vi "nanocal -- nuclear schottky fit V8.vi"() -> ()   [LabVIEW 2021] (continued)
          }
          frame "action: update state of selectors" {
            w1061 = T1[] [enum."T (K)", enum."B (T)", enum."θ (deg)", enum."side (S|R)"] items=["ζ", "τ1", "τS", "τN", "τC", "κ0", "m1", "m2", "m3", "T (K)", "B (T)", "θ (deg)", "side (S|R)", "set of (B|T)", "Re(offset)", "Im(offset)", "στ1", "στ1-", "στ1+", "στS", "στS-", "στS+", "στN", "στN-", "στN+", "τ11", "τ12", "τ21", "τ22", "τN1", "τN2", "σηlogτ1", "σηlogτS", "σηlogτN", "σlogτ1", "σlogτS", "σlogτN", "σητ1", "σητS", "σητN", "noiseT"]  # selector fields
            n504 = local read "what?"() -> (w1057:T6)
            n505 = Unbundle By Name(w1057) -> ("side (8S|4R)"=w1056:i64, "ignore side !"=w1055:bool, "lookup.side lookup"=w1054:map{i32, dbl}, "T (K)"=w1051:dbl, "ignore T !"=w1053:bool, "lookup.T lookup"=w1052:map{i32, dbl}, "B (T)"=w1048:dbl, "ignore B !"=w1050:bool, "lookup.B lookup"=w1049:map{i32, dbl}, "θ (∘)"=w1046:dbl, "ignore θ !"=w1045:bool, "lookup.θ lookup"=w1047:map{i32, dbl}, "set (1T|2B)"=w1042:i32, "ignore set of !"=w1043:bool, "lookup.set of lookup"=w1044:map{i32, dbl})
            n506 = local read "new selector names"() -> (w1064:map{T1, map{T14, string}})
            n507 = Look In Map(map=w1054, key=w1056) -> (value=w1060:dbl)  [unwired: 1 in, 1 out]
            n508 = node(w1055, w1060) -> (w1081:map{bool, dbl})
            n509 = Look In Map(map=w1052, key=w1051) -> (value=w1080:dbl)  [unwired: 1 in, 1 out]
            n510 = Look In Map(map=w1049, key=w1048) -> (value=w1076:dbl)  [unwired: 1 in, 1 out]
            n511 = node(w1053, w1080) -> (w1078:map{bool, dbl})
            n512 = node(w1050, w1076) -> (w1075:map{bool, dbl})
            n513 = Look In Map(map=w1047, key=w1046) -> (value=w1074:dbl)  [unwired: 1 in, 1 out]
            n514 = node(w1045, w1074) -> (w1072:map{bool, dbl})
            n515 = Look In Map(map=w1044, key=w1042) -> (value=w1071:dbl)  [unwired: 1 in, 1 out]
            n516 = node(w1043, w1071) -> (w1069:map{bool, dbl})
            n517 = local read "side map from NUM"() -> (w1058:map{i32, T9})
            n518 = node(3-lorentzian-parameters."side (S|R)" ("Plost: sweep window"), w1081, 3-lorentzian-parameters."T (K)" ("Plost: sweep window"), w1078, 3-lorentzian-parameters."B (T)" ("Plost: sweep window"), w1075, 3-lorentzian-parameters."θ (deg)" ("Plost: sweep window"), w1072, 3-lorentzian-parameters."set of (B|T)" ("Plost: sweep window"), w1069) -> (w1041:map{T1, map{bool, dbl}})
            "state of all selectors" <- w1041
            n519 = for {
              tunnel: w1064 -> [w1086]
              shift-right: [w1089] -> w1062
              shift-left: "_" ("event data") -> [w1088]
              tunnel: w1061 -> [w1085] mode=indexing
              tunnel: w1041 -> [w1083]
              n520 = Look In Map(map=w1083, key=w1085) -> (value=w1091:map{bool, dbl})  [unwired: 1 in, 1 out]
              n521 = Look In Map(map=w1086, key=w1085) -> (value=w1084:map{T14, string})  [unwired: 1 in, 1 out]
              n522 = for {
                tunnel: w1091 -> [w1106] mode=indexing
                tunnel: [w1105] -> w1090
                tunnel: [w1104] -> w1087
                n523 = Unbundle(w1106) -> ("ignore side !"=w1105:bool, "number OUT"=w1104:dbl)
              }
              n524 = case shown="False" w1090 {
                tunnel: [w1102 w1103] -> w1089
                tunnel: w1088 -> [w1101 w1103]
                tunnel: w1087 -> [w1098 _]
                tunnel: w1084 -> [w1094 _]
                frame False {
                  n525 = Look In Map(map=w1094, key=nameformattingitem."units") -> (value=w1095:string)  [unwired: 1 in, 1 out]
                  n526 = Look In Map(map=w1094, key=nameformattingitem."prec") -> (value=w1092:string)  [unwired: 1 in, 1 out]
                  n527 = Format Value(format string=w1092, value (0)=w1098) -> (output string=w1097:string)  [unwired: 1 in]
                  n528 = Concatenate Strings(w1101, "_" ("event data"), w1097, w1095, "_" ("event data")) -> (w1102:string)
                }
                frame True {
                }
              }
            }
            "state of all selectors string" <- w1062
            n529 = Look In Map(map=w1058, key=w1060) -> (value=w1059:T9)  [unwired: 1 in, 1 out]
            n530 = local write "side"(w1059) -> ()
            n531 = Generate User Event(user event=w1065, event data cluster="action: replot colors" ("event data")) -> (user event out=w1066:refnum<user-event>)  [unwired: 2 in, 1 out]
            n532 = Generate User Event(user event=w1066, event data cluster="action: update constrained file selector" ("event data")) -> ()  [unwired: 2 in, 2 out]
          }
          frame "action: copy from math" {
            w1107 = map{T1, dbl} {}  # Size: 0
            w1125 = map{T1, bool} {}  # Size: 0
            n533 = local read "defaults selector"() -> (w1124:T5)
            n534 = local read "mathematica thing"() -> (w1130:map{string, map{T1, dbl}})
            n535 = for {
              shift-right: [w1148] -> w1123
              shift-left: w1125 -> [w1149]
              tunnel: w1124 -> [w1147] mode=indexing
              n536 = Unbundle(w1147) -> ("Plost: sweep window"=w1146:T1, "used default"=w1145:bool)
              n537 = Insert Into Map(map in=w1149, key=w1146, value=w1145) -> (map out=w1148:map{T1, bool})  [unwired: 2 out]
            }
            n538 = case shown="True" "overwrite \noffset" {
              selector: "overwrite \noffset" -> [w1139 w1141]
              tunnel: w1122 -> [w1140 w1144]
              tunnel: [w1140 w1143] -> w1115
              tunnel: w1117 -> [_ w1142]
              tunnel: [w1139 w1141] -> w1108
              frame False {
              }
              frame True {
                n539 = Build Array (concatenate)(w1144, w1142) -> (w1143:T1[])
              }
            }
            n540 = local read "key"() -> (w1129:string)
            n541 = local read "parameter map"() -> (w1120:map{T1, dbl})
            n542 = case shown="True" "overwrite noiseT" {
              selector: "overwrite noiseT" -> [w1131 w1133]
              tunnel: w1115 -> [w1132 w1136]
              tunnel: [w1132 w1135] -> w1116
              tunnel: w1114 -> [_ w1134]
              tunnel: [w1131 w1133] -> w1112
              frame False {
              }
              frame True {
                n543 = Build Array (concatenate)(w1136, w1134) -> (w1135:T1[])
              }
            }
            n544 = Look In Map(map=w1130, key=w1129) -> (key not found?=w1127:bool, value=w1128:map{T1, dbl})  [unwired: 1 in]
            n545 = case shown="False" w1127 {
              tunnel: w1128 -> [w1163 _]
              tunnel: w1123 -> [w1161 _]
              tunnel: w1116 -> [w1162 _]
              tunnel: w1108 -> [w1160 w1206]
              tunnel: [w1159 w1206] -> w1111
              tunnel: w1120 -> [w1158 _]
              tunnel: w1118 -> [w1157 _]
              tunnel: w1112 -> [w1154 w1205]
              tunnel: [w1153 w1205] -> w1110
              tunnel: w1107 -> [w1151 _]
              frame False {
                # "the order of numbers \nMUST corrspond to order\nin the \"parameter\" array"
                n546 = for {
                  tunnel: w1163 -> [w1197]
                  tunnel: w1162 -> [w1187] mode=indexing
                  tunnel: w1161 -> [w1196]
                  shift-right: [w1191] -> w1152
                  shift-left: w1158 -> [w1192]
                  shift-right: [w1188] -> w1150
                  shift-left: w1151 -> [w1189]
                  n547 = Look In Map(map=w1196, key=w1187, default value=FALSE) -> (value=w1195:bool)  [unwired: 1 out]
                  n548 = Look In Map(map=w1197, key=w1187, default value=0.0) -> (value=w1194:dbl)  [unwired: 1 out]
                  n549 = case shown="True" w1195 {
                    tunnel: w1194 -> [w1200 _]
                    tunnel: w1187 -> [_ w1202]
                    tunnel: [w1200 w1201] -> w1186
                    frame False {
                    }
                    frame True {
                      n550 = local read "T (K)"() -> (w1204:dbl)
                      n551 = call "nanocal -- defaut parameter manager -- V1.vi"("action"=nanocal_--_defaut_parameter_manager_action--_V1."get logarithmic interp", "T"=w1204, "what"=w1202) -> ("number"=w1201:dbl)  [unwired: 8 in]
                    }
                  }
                  n552 = Insert Into Map(map in=w1189, key=w1187, value=w1186) -> (map out=w1188:map{T1, dbl})  [unwired: 2 out]
                  n553 = in-place {
                    in-place-border: w1186 -> [w1199]
                    in-place-border: LVMapReplaceAction."Modify Entry only if found" ("action") -> [w1198]
                    n554 = in-place-map #5(w1192, w1187) -> ()  [unwired: 1 in, 2 out]
                    n555 = in-place-map #5(w1199, w1198) -> (w1191:map{T1, dbl})  [unwired: 2 out]
                  }
                }
                n556 = case shown="True" w1154 {
                  selector: w1154 -> [w1164 w1170]
                  tunnel: [w1164 w1170] -> w1153
                  tunnel: w1150 -> [_ w1168]
                  frame False {
                  }
                  frame True {
                    n557 = local read "errors&stuff"() -> (w1167:T10)
                    n558 = Look In Map(map=w1168, key=3-lorentzian-parameters."noiseT" ("x")) -> (value=w1166:dbl)  [unwired: 1 in, 1 out]
                    n559 = in-place {
                      in-place-border: w1166 -> [w1171]
                      n560 = in-place-cluster #6(w1167) -> ()  [unwired: 1 out]
                      n561 = in-place-cluster #6("noise T"=w1171) -> (w1165:T10)
                    }
                    n562 = local write "errors&stuff"(w1165) -> ()
                  }
                }
                n563 = case shown="True" w1160 {
                  selector: w1160 -> [w1177 w1184]
                  tunnel: [w1177 w1184] -> w1159
                  tunnel: w1150 -> [_ w1183]
                  frame False {
                  }
                  frame True {
                    n564 = Look In Map(map=w1183, key=3-lorentzian-parameters."Im(offset)" ("x")) -> (value=w1179:dbl)  [unwired: 1 in, 1 out]
                    n565 = Look In Map(map=w1183, key=3-lorentzian-parameters."Re(offset)" ("x")) -> (value=w1180:dbl)  [unwired: 1 in, 1 out]
                    n566 = Bundle("number OUT"=w1180, "number OUT"=w1179) -> (w1178:cluster{"number OUT":dbl, "number OUT":dbl})  [unwired: 1 in]
                    n567 = local write "offset Re\noffset Im"(w1178) -> ()
                  }
                }
                n568 = flat-sequence {
                  tunnel: w1152 -> [w1172]
                  tunnel: w1157 -> [w1176]
                  tunnel: "interface: update list from parameter map" ("event data") -> [w1175]
                  tunnel: "interface: update curvature plot" ("event data") -> [w1173]
                  frame #0 {
                    n569 = local write "parameter map"(w1172) -> ()
                  }
                  frame #1 {
                    n570 = Generate User Event(user event=w1176, event data cluster=w1175) -> (user event out=w1174:refnum<user-event>)  [unwired: 2 in, 1 out]
                    n571 = Generate User Event(user event=w1174, event data cluster=w1173) -> ()  [unwired: 2 in, 2 out]
                  }
                }
              }
              frame True {
              }
            }
            n572 = Or(x=w1111, y=w1110) -> (x .or. y?=w1109:bool)
            n573 = case shown="True" w1109 {
              tunnel: ["action: new sweep" ("event data") "action: read from file" ("event data")] -> w1119
              frame False {
              }
              frame True {
              }
            }
            n574 = Generate User Event(user event=w1126, event data cluster=w1119) -> ()  [unwired: 2 in, 2 out]
          }
          frame "action: copy to math" {
            n575 = local read "newton parameters"() -> (w1228:T2)
            n576 = local read "error weights"() -> (w1227:T4)
            n577 = local read "parameter map"() -> (w1217:map{T1, dbl})
            n578 = local read "errors&stuff"() -> (w1211:T10)
            n579 = call "nanocal -- publish -- freq scan V2.vi"("publisher action"=publisher_action."get") -> ("data"=w1218:T21)  [unwired: 7 in, 3 out]
            n580 = Bundle By Name(cluster=w1228, "weighting"=w1227) -> (w1219:T2)
            n581 = Generate User Event(user event=w1241, event data cluster="action: replot colors" ("event data")) -> ()  [unwired: 2 in, 2 out]
            n582 = call "nanocal -- generate 3D curvature ellipsoid --  V5.vi"("parameter keys IN"=w1216, "parameter tensor order IN"=w1215, "parameters IN"=w1217, "data IN"=w1218, "errors IN"=w1211, "newton parameters"=w1219) -> ("errors pair OUT"=w1209:T10)  [unwired: 9 in]
            n583 = Build Array (concatenate)(w1220, w1222, w1208, w1207) -> (w1221:T1[])
            n584 = Unbundle By Name(w1209) -> ("pars & errors"=w1223:map{T1, dbl})
            n585 = local write "errors&stuff"(w1209) -> ()
            n586 = local read "offset Re\noffset Im"() -> (w1231:cluster{"Numeric":dbl, "Numeric":dbl})
            n587 = local read "θ (deg)"() -> (w1235:dbl)
            n588 = for {
              tunnel: w1222 -> [w1245] mode=indexing
              shift-right: [w1246] -> _
              shift-left: w1223 -> [w1246]
              tunnel: [w1244] -> w1225 mode=indexing
              n589 = Look In Map(map=w1246, key=w1245, default value=0.0) -> (value=w1244:dbl)  [unwired: 1 out]
            }
            n590 = local read "T (K)"() -> (w1237:dbl)
            n591 = local read "B (T)"() -> (w1236:dbl)
            n592 = Unbundle(w1231) -> ("Numeric"=w1214:dbl, "Numeric"=w1213:dbl)
            n593 = Unbundle By Name(w1209) -> ("noise T"=w1210:dbl)
            n594 = local read "parameter map"() -> (w1230:map{T1, dbl})
            n595 = Build Array(w1214, w1213) -> (w1212:dbl[])
            n596 = Build Array(w1237, w1236, w1235) -> (w1226:dbl[])
            n597 = Build Array (concatenate)(w1226, w1225, w1212, w1210) -> (w1224:dbl[])
            n598 = for {
              tunnel: w1224 -> [w1247] mode=indexing
              tunnel: w1221 -> [w1248] mode=indexing
              shift-right: [w1249] -> w1234
              shift-left: w1230 -> [w1250]
              n599 = Insert Into Map(map in=w1250, key=w1248, value=w1247) -> (map out=w1249:map{T1, dbl})  [unwired: 2 out]
            }
            n600 = local read "mathematica thing"() -> (w1240:map{string, map{T1, dbl}})
            n601 = local read "key"() -> (w1239:string)
            n602 = call "3-lorentzian-heat-response -- V4.vi"("action"=3-lorentzian-heat-response_action."calc m1m2m3", "Map IN"=w1234) -> ("Map OUT"=w1233:map{T1, dbl})  [unwired: 7 in, 2 out]
            n603 = in-place {
              in-place-border: w1233 -> [w1251]
              n604 = in-place-map #7(w1240, w1239) -> (w1254:map{T1, dbl})  [unwired: 1 in, 1 out]
              n605 = for {
                tunnel: w1251 -> [w1256] mode=indexing
                shift-right: [w1259] -> w1253
                shift-left: w1254 -> [w1260]
                shift-right: [w1258] -> _
                shift-left: w1251 -> [w1258]
                n606 = Unbundle(w1256) -> ("X selector"=w1255:T1)  [unwired: 1 out]
                n607 = Look In Map(map=w1258, key=w1255) -> (value=w1257:dbl)  [unwired: 1 in, 1 out]
                n608 = Insert Into Map(map in=w1260, key=w1255, value=w1257) -> (map out=w1259:map{T1, dbl})  [unwired: 2 out]
              }
              n609 = in-place-map #7(w1253, LVMapReplaceAction."Modify Entry only if found" ("action")) -> (w1238:map{string, map{T1, dbl}})  [unwired: 2 out]
            }
            n610 = local write "mathematica thing"(w1238) -> ()
          }
          frame "action: exit" {
          }
          frame "action: read from file" {
            n611 = local read "Read from file"() -> (w1269:path)
            n612 = Unbundle("offset Re\noffset Im") -> ("Numeric"=w1295:dbl, "Numeric"=w1294:dbl)
            n613 = Re/Im To Complex(1:w1294, 2:w1295) -> (0:w1282:cdb)
            n614 = call "file - read-write - list of lines-V2.vi"("read/write control"=file_--_read-write_control."read", "file path"=w1269) -> ("header OUT"=w1279:string, "list of lines OUT"=w1281:string[], "filename out"=w1309:string)  [unwired: 7 in]
            n615 = local read "cursor x selector"() -> (w1292:map{T1, dbl})
            n616 = call "filename-manage.vi"("filename-action"=filename-action."get name", "file name IN"=w1309) -> ("string OUT"=w1278:string)  [unwired: 7 in, 2 out]
            n617 = call "filename-manage.vi"("filename-action"=filename-action."get T", "file name IN"=w1278) -> ("number OUT"=w1291:dbl, "filename OUT"=w1306:string)  [unwired: 7 in, 1 out]
            "T (K)" <- w1291
            n618 = case shown="\"raw nanocal\"" "data file formatting" {
              tunnel: [w1318 w1345 w1394 w1421] -> w1303
              tunnel: [w1317 w1344 w1393 w1420] -> w1297
              tunnel: w1282 -> [w1316 w1339 w1389 w1410]
              tunnel: w1281 -> [w1319 w1353 w1388 w1409]
              tunnel: w1279 -> [_ w1354 _ _]
              tunnel: w1278 -> [_ w1351 _ _]
              tunnel: w1269 -> [_ w1352 _ _]
              tunnel: "side" -> [_ w1350 _ _]
              tunnel: "toggle generate labview files" -> [_ w1348 _ _]
              tunnel: "apply RC transform" -> [_ w1332 _ _]
              frame "as is", Default {
                n619 = for {
                  tunnel: w1319 -> [w1330] mode=indexing
                  tunnel: [w1325] -> w1320 mode=indexing if=w1321
                  tunnel: [w1324] -> w1318 mode=indexing if=w1321
                  w1326 = 0.0
                  n620 = Scan From String(format string="%f%f%f", input string=w1330, initial scan location=u32 0, default 1=w1326, default 2=w1326, default 3=w1326) -> (offset past scan=w1322:u32, output 1=w1324:dbl, output 2=w1328:dbl, output 3=w1327:dbl)  [unwired: 1 in, 2 out]
                  n621 = Greater Than 0?(x=w1322) -> (x > 0?=w1321:bool)
                  n622 = Re/Im To Complex(1:w1327, 2:w1328) -> (0:w1325:cdb)
                }
                n623 = Subtract(x=w1320, y=w1316) -> (x-y=w1317:cdb[])
              }
              frame "raw nanocal" {
                (unwired) array_--_freq-voltage_transformations_action."add -ω" ("freq voltage action")
                w1347 = T29[] [enum."add -ω", enum."sort ω", enum."select |ω|<max"] items=["as is", "add -ω", "sort ω", "2 x ω", "R-phase(deg) to Re-Im", "select ω>0", "labview file str", "select |ω|<max", "apply RC transform", "subtract background"]
                n624 = case shown="\"ref\"" w1350 {
                  tunnel: [nanocal_raw_file_manage_action_V1."read S side" ("action") nanocal_raw_file_manage_action_V1."read R side" ("action")] -> w1349
                  frame "sam", Default {
                  }
                  frame "ref" {
                  }
                }
                n625 = call "nanocal_raw_file_manage_V1.vi"("action"=w1349, "list of lines IN"=w1353, "header IN"=w1354) -> ("z (K/W)  OUT"=w1338:cdb[], "f (Hz) OUT"=w1341:dbl[], "correct temperature"=→"correct temperature":dbl)  [unwired: 5 in, 1 out]
                n626 = call "array -- freq-voltage transformations.vi"("number"=w1339, "freq voltage action"=array_--_freq-voltage_transformations_action."subtract background", "z In"=w1338, "ω IN"=w1341) -> ("z out"=w1336:cdb[], "ω out"=w1340:dbl[])  [unwired: 4 in, 2 out]
                n627 = case shown="True" w1332 {
                  tunnel: w1340 -> [w1356 w1363]
                  tunnel: [w1356 w1362] -> w1337
                  tunnel: w1336 -> [w1355 w1361]
                  tunnel: [w1355 w1360] -> w1335
                  tunnel: "tau" -> [_ w1359]
                  tunnel: array_--_freq-voltage_transformations_action."apply RC transform" ("freq voltage action") -> [_ w1358]
                  tunnel: "alpha" -> [_ w1357]
                  frame False {
                  }
                  frame True {
                    n628 = call "array -- freq-voltage transformations.vi"("number"=w1359, "freq voltage action"=w1358, "alpha"=w1357, "z In"=w1361, "ω IN"=w1363) -> ("z out"=w1360:cdb[], "ω out"=w1362:dbl[])  [unwired: 3 in, 2 out]
                  }
                }
                n629 = for {
                  shift-right: [w1367] -> w1345
                  shift-left: w1337 -> [w1368]
                  shift-right: [w1366] -> w1344
                  shift-left: w1335 -> [w1369]
                  tunnel: w1347 -> [w1365] mode=indexing
                  tunnel: "|ω| < limit (Hz)" -> [w1364]
                  n630 = call "array -- freq-voltage transformations.vi"("number"=w1364, "freq voltage action"=w1365, "z In"=w1369, "ω IN"=w1368) -> ("z out"=w1366:cdb[], "ω out"=w1367:dbl[])  [unwired: 4 in, 2 out]
                }
                n631 = case shown="True" w1348 {
                  tunnel: w1352 -> [_ w1381]
                  tunnel: w1351 -> [_ w1385]
                  tunnel: w1345 -> [_ w1377]
                  tunnel: w1344 -> [_ w1376]
                  frame False {
                  }
                  frame True {
                    n632 = call "filename-manage.vi"("filename-action"=filename-action."get basename", "file name IN"=w1385) -> ("string OUT"=w1383:string)  [unwired: 7 in, 2 out]
                    n633 = Strip Path(path=w1381) -> (stripped path=w1380:path)  [unwired: 1 out]
                    n634 = Concatenate Strings(w1383, "_labview_.dat") -> (w1372:string)
                    n635 = call "array -- freq-voltage transformations.vi"("freq voltage action"=array_--_freq-voltage_transformations_action."labview file str", "z In"=w1376, "ω IN"=w1377) -> ("lines out"=w1374:string[], "header OUT"=w1375:string)  [unwired: 5 in, 2 out]
                    n636 = Build Path(base path=w1380, name or relative path=w1372) -> (appended path=w1379:path)
                    n637 = call "file - read-write - list of lines-V2.vi"("read/write control"=file_--_read-write_control."write all", "header IN"=w1375, "list of lines IN"=w1374, "file path"=w1379) -> ()  [unwired: 5 in, 3 out]
                  }
                }
              }
              frame "add - ω" {
                n638 = for {
                  tunnel: w1388 -> [w1406] mode=indexing
                  tunnel: [w1401] -> w1390 mode=indexing if=w1397
                  tunnel: [w1400] -> w1386 mode=indexing if=w1397
                  w1402 = 0.0
                  n639 = Scan From String(format string="%f%f%f", input string=w1406, initial scan location=u32 0, default 1=w1402, default 2=w1402, default 3=w1402) -> (offset past scan=w1398:u32, output 1=w1400:dbl, output 2=w1404:dbl, output 3=w1403:dbl)  [unwired: 1 in, 2 out]
                  n640 = Greater Than 0?(x=w1398) -> (x > 0?=w1397:bool)
                  n641 = Re/Im To Complex(1:w1403, 2:w1404) -> (0:w1401:cdb)
                }
                n642 = Subtract(x=w1390, y=w1389) -> (x-y=w1387:cdb[])
                n643 = call "array -- freq-voltage transformations.vi"("freq voltage action"=array_--_freq-voltage_transformations_action."add -ω", "z In"=w1387, "ω IN"=w1386) -> ("z out"=w1395:cdb[], "ω out"=w1396:dbl[])  [unwired: 5 in, 2 out]
                n644 = call "array -- freq-voltage transformations.vi"("freq voltage action"=array_--_freq-voltage_transformations_action."sort ω", "z In"=w1395, "ω IN"=w1396) -> ("z out"=w1393:cdb[], "ω out"=w1394:dbl[])  [unwired: 5 in, 2 out]
              }
              frame "full rydh" {
                n645 = for {
                  tunnel: w1409 -> [w1433] mode=indexing
                  tunnel: [w1428] -> w1411 mode=indexing if=w1424
                  tunnel: [w1427] -> w1407 mode=indexing if=w1424
                  w1429 = 0.0
                  n646 = Scan From String(format string="%f%f%f", input string=w1433, initial scan location=u32 0, default 1=w1429, default 2=w1429, default 3=w1429) -> (offset past scan=w1425:u32, output 1=w1427:dbl, output 2=w1431:dbl, output 3=w1430:dbl)  [unwired: 1 in, 2 out]
                  n647 = Greater Than 0?(x=w1425) -> (x > 0?=w1424:bool)
                  n648 = Re/Im To Complex(1:w1430, 2:w1431) -> (0:w1428:cdb)
                }
                n649 = Subtract(x=w1411, y=w1410) -> (x-y=w1408:cdb[])
                n650 = call "array -- freq-voltage transformations.vi"("freq voltage action"=array_--_freq-voltage_transformations_action."2 x ω", "z In"=w1408, "ω IN"=w1407) -> ("z out"=w1415:cdb[], "ω out"=w1417:dbl[])  [unwired: 5 in, 2 out]
                n651 = call "array -- freq-voltage transformations.vi"("freq voltage action"=array_--_freq-voltage_transformations_action."R-phase(deg) to Re-Im", "z In"=w1415, "ω IN"=w1417) -> ("z out"=w1414:cdb[], "ω out"=w1416:dbl[])  [unwired: 5 in, 2 out]
                n652 = call "array -- freq-voltage transformations.vi"("freq voltage action"=array_--_freq-voltage_transformations_action."add -ω", "z In"=w1414, "ω IN"=w1416) -> ("z out"=w1422:cdb[], "ω out"=w1423:dbl[])  [unwired: 5 in, 2 out]
                n653 = call "array -- freq-voltage transformations.vi"("freq voltage action"=array_--_freq-voltage_transformations_action."sort ω", "z In"=w1422, "ω IN"=w1423) -> ("z out"=w1420:cdb[], "ω out"=w1421:dbl[])  [unwired: 5 in, 2 out]
              }
            }
            n654 = Insert Into Map(map in=w1292, key=3-lorentzian-parameters."T (K)" ("Plost: sweep window"), value=w1291) -> (map out=w1290:map{T1, dbl})  [unwired: 2 out]
            n655 = call "filename-manage.vi"("filename-action"=filename-action."get deg", "file name IN"=w1306) -> ("number OUT"=w1287:dbl, "filename OUT"=w1273:string)  [unwired: 7 in, 1 out]
            "θ (deg)" <- w1287
            n656 = Insert Into Map(map in=w1290, key=3-lorentzian-parameters."θ (deg)" ("Plost: sweep window"), value=w1287) -> (map out=w1289:map{T1, dbl})  [unwired: 2 out]
            n657 = call "filename-manage.vi"("filename-action"=filename-action."get B", "file name IN"=w1273) -> ("number OUT"=w1286:dbl, "filename OUT"=w1272:string)  [unwired: 7 in, 1 out]
            "B (T)" <- w1286
            n658 = Insert Into Map(map in=w1289, key=3-lorentzian-parameters."B (T)" ("Plost: sweep window"), value=w1286) -> (map out=w1288:map{T1, dbl})  [unwired: 2 out]
            n659 = local read "side map to STR"() -> (w1271:map{T9, string})
            n660 = local write "cursor x selector"(w1288) -> ()
            n661 = call "filename-manage.vi"("filename-action"=filename-action."getIDStock", "file name IN"=w1272) -> ("string OUT"=w1276:string)  [unwired: 7 in, 2 out]
            "file IDS" <- w1276
            n662 = Look In Map(map=w1271, key="side") -> (value=w1277:string)  [unwired: 1 in, 1 out]
            n663 = Concatenate Strings(w1276, w1277) -> (→"key":string)
            n664 = local read "folder"() -> (w1268:path)
            n665 = Build Path(base path=w1268, name or relative path=path "PLOTME.dat") -> (appended path=w1266:path)
            n666 = call "filter - complex - four.vi"("omega (Hz) in"=w1303, "z in"=w1297, "span"="cspan") -> ("omega out"=w1302:dbl[], "z out"=w1301:cdb[], "dz/domega out"=w1300:cdb[])  [unwired: 9 in, 5 out]
            n667 = call <vilib>:"Check if File or Folder Exists.vi"("path"=w1266) -> ("file or folder exists?"=w1265:bool, "dup path"=w1264:path)  [unwired: 8 in, 1 out]
            n668 = call "nanocal -- publish -- freq scan V2.vi"("publisher action"=publisher_action."set", "dz/dω IN (V)"=w1300, "z IN (V)"=w1301, "ω IN (Hz)"=w1302) -> ()  [unwired: 4 in, 4 out]
            n669 = case shown="True" w1265 {
              tunnel: w1264 -> [_ w1315]
              tunnel: [map{string, dbl[]} {} ("waves OUT") w1314] -> w1263
              frame False {
              }
              frame True {
                n670 = call "read waves - -V1.vi"("file path"=w1315) -> ("waves OUT"=w1314:map{string, dbl[]})  [unwired: 10 in]
              }
            }
            n671 = Generate User Event(user event=w1310, event data cluster="action: new sweep" ("event data")) -> ()  [unwired: 2 in, 2 out]
            n672 = local write "plotme waves"(w1263) -> ()
          }
          frame "action: save freq scan" {
            n673 = local read "Freq sweep name template"() -> (w1439:T8)
            n674 = call "MFLI -- publish -- freq scan.vi"("publisher action"=publisher_action."get") -> ("Voltage out (V)"=w1435:cdb[], "Freq out (Hz)"=w1436:dbl[])  [unwired: 9 in]
            n675 = call "filename-manage.vi"("filename pattern"=w1439, "filename-action"=filename-action."uniquenum", "folder IN"="Save folder", "file name IN"="freq sweep file name") -> ("filename OUT"=w1438:string)  [unwired: 5 in, 2 out]
            n676 = call "KM_appendline -- freq sweep.vi"("freq"=w1436, "Vout(V)"=w1435, "Save frequency scan"="Save folder", "read/write control"=KM_file_--_read-write_control."append one line", "name or relative path"=w1438) -> ()  [unwired: 15 in]
            n677 = local write "freq sweep file name"(w1438) -> ()
          }
          frame "void", Default {
          }
        }
      }
    }
  }
  n678 = while "interface events" {
    tunnel: w18 -> [w1447]
    tunnel: w45 -> [w1446]
    tunnel: w42 -> [w1445]
    tunnel: w19 -> [w1444]
    stop <- FALSE stop-if-true
    n679 = event shown="[10] \"alpha\", \"|ω| < limit (Hz)\", \"cspan\", \"tau\", \"apply RC transform\", \"offset Re offset Im\": Value Change" {
      selector: _ -> [_ _ _ _ _ _ _ _ _ _ _ _ _ _ _ _ _ _ _ _ _ _ _ _ _ _]
      dyn-events: _ -> [_ _ _ _ _ _ _ _ _ _ _ _ _ _ _ _ _ _ _ _ _ _ _ _ _ _]
      timeout: _ -> [_ _ _ _ _ _ _ _ _ _ _ _ _ _ _ _ _ _ _ _ _ _ _ _ _ _]
      tunnel: w1447 -> [w1448 _ w1461 w1485 _ w1510 w1516 _ w1520 w1522 w1524 w1527 w1533 _ w1627 w1648 w1668 w1670 w1674 w1677 w1680 w1683 w1691 w1695 w1697 w1700]
      tunnel: [_ _ _ _ _ _ _ _ "load! :l" _ _ _ _ _ _ _ _ _ _ _ _ _ _ _ _ _] -> _
      tunnel: [_ _ _ _ _ "go / pause!" _ _ _ _ _ "parse! :p" _ _ _ _ "Math→τ! :q" _ "τ→Math! :p" "Math→ string OUT! :s" "generate empty string from filelist !" "string IN → Math! :~" _ _ "plot landscape!" _] -> _
      tunnel: w1446 -> [_ w1452 _ _ w1487 _ _ _ _ _ _ _ w1529 _ _ _ _ _ _ _ _ _ _ _ _ _]
      tunnel: w1445 -> [_ _ _ _ _ _ _ _ _ _ _ _ _ _ w1635 w1656 _ _ _ _ _ _ _ _ _ _]
      tunnel: [_ _ _ _ _ _ _ _ _ "Read from file" _ _ _ _ _ _ _ _ _ _ _ _ _ _ _ _] -> _
      tunnel: [_ _ _ _ _ _ _ _ _ _ _ _ _ _ _ _ _ "load defaults" _ _ _ _ _ _ _ _] -> _
      tunnel: w1444 -> [_ _ w1463 _ _ _ _ _ _ _ _ _ _ w1622 w1625 w1646 _ _ _ _ _ _ _ _ _ _]
      event "Plot: circles": Cursor Move {
        n680 = event-data() -> ("CursIdx"=w1449:i32)  [unwired: 1 in]
        n681 = case shown="0..2" w1449 {
          tunnel: w1448 -> [w1451 _]
          frame 0..2 {
            w1450 = "action: fit"  # action
            n682 = Generate User Event(user event=w1451, event data cluster=w1450) -> ()  [unwired: 2 in, 2 out]
          }
          frame 3..5, Default {
          }
        }
      }
      event "scale gauge: Plot: circles": Value Change {
        n683 = event-data() -> ()  [unwired: 1 in, 1 out]
        n684 = local read "scale gauge: Plot: circles"() -> (w1458:dbl)
        n685 = Multiply(x=w1458, y=0.3) -> (x*y=w1459:dbl)
        n686 = Bundle By Name(cluster=T35 {"window y"=0.0021014740628288917, "center x"=44850.89441339177, "center y"=2.5658109925320947, "window x"=17480.201988350764} ("window IN"), "window x"=w1458, "window y"=w1458, "center x"=w1459, "center y"=0.0) -> (w1457:T35)
        n687 = call "replace cursor - plot ref - V2.vi"("Plot ref in"=w1452, "window IN"=w1457, "cursor action"=cursor_action."zoom to win") -> ()  [unwired: 13 in, 4 out]
      }
      event "ζ", "T1", "τS", "τN", "τC", "κ0": Value Change {
        w1464 = T1[] [enum."ζ", enum."τ1", enum."τS", enum."τN", enum."τC", enum."κ0"] items=["ζ", "τ1", "τS", "τN", "τC", "κ0", "m1", "m2", "m3", "T (K)", "B (T)", "θ (deg)", "side (S|R)", "set of (B|T)", "Re(offset)", "Im(offset)", "στ1", "στ1-", "στ1+", "στS", "στS-", "στS+", "στN", "στN-", "στN+", "τ11", "τ12", "τ21", "τ22", "τN1", "τN2", "σηlogτ1", "σηlogτS", "σηlogτN", "σlogτ1", "σlogτS", "σlogτN", "σητ1", "σητS", "σητN", "noiseT"]
        n688 = event-data() -> ()  [unwired: 1 in, 1 out]
        n689 = local read "τN"() -> (w1470:dbl)
        n690 = local read "τC"() -> (w1469:dbl)
        n691 = local read "κ0"() -> (w1468:dbl)
        n692 = local read "T1"() -> (w1472:dbl)
        n693 = local read "τS"() -> (w1471:dbl)
        n694 = local read "ζ"() -> (w1473:dbl)
        n695 = local read "parameter map"() -> (w1465:map{T1, dbl})
        n696 = Build Array(w1473, w1472, w1471, w1470, w1469, w1468) -> (w1467:dbl[])
        n697 = for {
          tunnel: w1464 -> [w1479] mode=indexing
          shift-right: [w1484] -> _
          shift-left: w1467 -> [w1484]
          shift-right: [w1481] -> w1466
          shift-left: w1465 -> [w1482]
          i -> [w1483]
          n698 = Index Array(array=w1484, index=w1483) -> (element=w1480:dbl)
          n699 = Insert Into Map(map in=w1482, key=w1479, value=w1480) -> (map out=w1481:map{T1, dbl})  [unwired: 2 out]
        }
        n700 = flat-sequence {
          tunnel: w1466 -> [w1474]
          tunnel: w1463 -> [w1478]
          tunnel: "interface: update color cursors" ("event data") -> [w1477]
          tunnel: w1461 -> [w1476]
          tunnel: "action: replot circles" ("event data") -> [w1475]
          frame #0 {
            n701 = local write "parameter map"(w1474) -> ()
          }
          frame #1 {
            n702 = Generate User Event(user event=w1476, event data cluster=w1475) -> ()  [unwired: 2 in, 2 out]
            n703 = Generate User Event(user event=w1478, event data cluster=w1477) -> ()  [unwired: 2 in, 2 out]
          }
        }
      }
      event Value Change {
        n704 = event-data() -> ()  [unwired: 1 in, 6 out]
        n705 = Generate User Event(user event=w1485, event data cluster="action: update enums" ("event data")) -> ()  [unwired: 2 in, 2 out]
      }
      event "ω0 (rad/sec)": Value Change {
        n706 = event-data() -> ()  [unwired: 1 in, 1 out]
        n707 = local read "parameter map"() -> (w1489:map{T1, dbl})
        n708 = call "nanocal -- publish -- freq scan V2.vi"("publisher action"=publisher_action."get") -> ("z out (V)"=w1507:cdb[], "ω out (Hz)"=w1502:dbl[])  [unwired: 7 in, 2 out]
        n709 = Divide(x="ω0 (rad/sec)", y=6.283185307179586) -> (x/y=w1500:dbl)
        n710 = call "3-lorentzian-heat-response -- V4.vi"("action"=3-lorentzian-heat-response_action."calc R", "Map IN"=w1489, "omega IN (rad/sec)"="ω0 (rad/sec)") -> ("Romega"=w1499:cdb)  [unwired: 6 in, 2 out]
        n711 = Threshold 1D Array(2:w1500, 3:w1502) -> (0:w1501:dbl)  [unwired: 1 in]
        n712 = Complex To Re/Im(x + iy=w1499) -> (x=w1497:dbl, y=w1498:dbl)
        n713 = Index Array(array=w1507, index=w1501) -> (element=w1504:cdb)
        n714 = call "replace cursor - plot ref - V2.vi"("Plot ref in"=w1487, "new X"=w1497, "new  Y"=w1498, "cursor index"=0, "cursor action"=cursor_action."write") -> ("Plot ref out"=w1503:refnum<vi>)  [unwired: 11 in, 3 out]
        n715 = Complex To Re/Im(x + iy=w1504) -> (x=w1505:dbl, y=w1506:dbl)
        n716 = call "replace cursor - plot ref - V2.vi"("Plot ref in"=w1503, "new X"=w1505, "new  Y"=w1506, "cursor index"=1, "cursor action"=cursor_action."write") -> ()  [unwired: 11 in, 4 out]
      }
      event "go / pause!": Value Change {
        n717 = event-data() -> ()  [unwired: 1 in, 1 out]
        n718 = local read "newton is active"() -> (w1508:bool)
        n719 = case shown="True" w1508 {
          tunnel: w1510 -> [_ w1515]
          tunnel: [FALSE TRUE] -> w1509
          frame True {
          }
          frame False {
            n720 = Generate User Event(user event=w1515, event data cluster="action: gradient step" ("event data")) -> ()  [unwired: 2 in, 2 out]
          }
        }
        n721 = local write "newton is active"(w1509) -> ()
      }
      event "what?": Value Change {
        n722 = event-data() -> ()  [unwired: 1 in, 1 out]
        n723 = Generate User Event(user event=w1516, event data cluster="action: update state of selectors" ("event data")) -> ()  [unwired: 2 in, 2 out]
      }
      event "Plot: circles": Cursor Release {
        n724 = event-data() -> ()  [unwired: 1 in, 1 out]
      }
      event "load! :l": Value Change {
        n725 = event-data() -> ()  [unwired: 1 in, 6 out]
        n726 = Generate User Event "action User Event"(user event=w1520, event data cluster="action: read from file" ("event data")) -> ()  [unwired: 2 in, 2 out]
      }
      event "Read from file": Value Change {
        n727 = event-data() -> ()  [unwired: 1 in, 6 out]
        n728 = Generate User Event ("action User Event")(user event=w1522, event data cluster="action: read from file" ("event data")) -> ()  [unwired: 2 in, 2 out]
      }
      event "alpha", "|ω| < limit (Hz)", "cspan", "tau", "apply RC transform", "offset Re\noffset Im": Value Change {
        n729 = event-data() -> ()  [unwired: 1 in, 6 out]
        n730 = Generate User Event "action User Event"(user event=w1524, event data cluster="action: read from file" ("event data")) -> ()  [unwired: 2 in, 2 out]
      }
      event "parse! :p": Value Change {
        n731 = event-data() -> ()  [unwired: 1 in, 6 out]
        n732 = Generate User Event "action User Event"(user event=w1527, event data cluster="action: parse string" ("event data")) -> ()  [unwired: 2 in, 2 out]
      }
      event Key Down {
        n733 = event-data() -> ("Char"=w1531:i16, "VKey"=w1534:T36)  [unwired: 1 in]
        n734 = Build Array(w1531) -> (w1532:i16[])
        n735 = Byte Array To String(unsigned byte array=w1532) -> (string=w1530:string)
        n736 = case shown="\"Up\"..\"Right\"" w1534 {
          selector: w1534 -> [_ _ _ _ _ w1617]
          tunnel: w1533 -> [w1537 _ w1611 _ _ _]
          tunnel: w1530 -> [w1536 _ _ _ _ _]
          tunnel: w1529 -> [w1535 _ _ _ _ w1616]
          frame "ASCII", Default {
            n737 = case shown="\"?\"" w1536 {
              selector: w1536 -> [_ _ _ _ _ _ _ w1560 w1570 _ _ _ _ w1590 _]
              tunnel: w1537 -> [_ _ w1538 w1540 w1542 w1546 _ _ _ _ w1581 w1584 w1586 w1588 w1609]
              tunnel: w1535 -> [_ _ _ _ _ _ w1556 _ _ _ _ _ _ _ _]
              frame "0", Default {
              }
              frame "a" {
              }
              frame "s" {
                n738 = Generate User Event(user event=w1538, event data cluster="action: write mathematica string" ("event data")) -> ()  [unwired: 2 in, 2 out]
              }
              frame "~" {
                n739 = Generate User Event(user event=w1540, event data cluster="action: read mathematica string" ("event data")) -> ()  [unwired: 2 in, 2 out]
              }
              frame "l" {
                n740 = Generate User Event(user event=w1542, event data cluster="action: read from file" ("event data")) -> ()  [unwired: 2 in, 2 out]
              }
              frame " " {
                n741 = local read "newton is active"() -> (w1545:bool)
                n742 = case shown="False" w1545 {
                  selector: w1545 -> [w1548 w1550]
                  tunnel: w1546 -> [_ w1552]
                  tunnel: [w1547 w1549] -> w1544
                  frame True {
                    n743 = Not(x=w1548) -> (.not. x?=w1547:bool)
                  }
                  frame False {
                    n744 = Generate User Event(user event=w1552, event data cluster="action: gradient step" ("event data")) -> ()  [unwired: 2 in, 2 out]
                    n745 = Not(x=w1550) -> (.not. x?=w1549:bool)
                  }
                }
                n746 = local write "newton is active"(w1544) -> ()
              }
              frame "?" {
                # "?"
                n747 = call "replace cursor - plot ref - V2.vi"("Plot ref in"=w1556, "cursor action"=cursor_action."zoom to win") -> ("Plot ref out"=w1555:refnum<vi>)  [unwired: 14 in, 3 out]
                n748 = call "replace cursor - plot ref - V2.vi"("Plot ref in"=w1555, "cursor action"=cursor_action."smart zoom out&aspect") -> ()  [unwired: 14 in, 4 out]
              }
              frame ",", "." {
                n749 = local read "newton parameters"() -> (w1558:T2)
                n750 = case shown="\".\"" w1560 {
                  tunnel: [0.7 1.0 1.5] -> w1559
                  frame "," {
                  }
                  frame "0", Default {
                  }
                  frame "." {
                  }
                }
                n751 = in-place {
                  in-place-border: w1559 -> [w1563]
                  n752 = in-place-cluster #8(w1558) -> ("PID-P"=w1561:dbl)
                  n753 = Multiply(x=w1563, y=w1561) -> (x*y=w1562:dbl)
                  n754 = in-place-cluster #8("PID-P"=w1562) -> (w1557:T2)
                }
                n755 = local write "newton parameters"(w1557) -> ()
              }
              frame "<", ">" {
                n756 = local read "newton parameters"() -> (w1568:T2)
                n757 = case shown="\"<\"" w1570 {
                  tunnel: [-5 0 5] -> w1569
                  frame "<" {
                  }
                  frame "0", Default {
                  }
                  frame ">" {
                  }
                }
                n758 = in-place {
                  in-place-border: w1569 -> [w1576]
                  n759 = in-place-cluster #9(w1568) -> ("PID-I"=w1575:i32)
                  n760 = Add(x=w1576, y=w1575) -> (x+y=w1574:i32)
                  n761 = In Range and Coerce(upper limit=100, x=w1574, lower limit=2) -> (coerced(x)=w1571:i32)  [unwired: 1 out]
                  n762 = in-place-cluster #9("PID-I"=w1571) -> (w1567:T2)
                }
                n763 = local write "newton parameters"(w1567) -> ()
              }
              frame "b" {
                n764 = local read "String"() -> (w1580:string)
                n765 = local write "backup string :b"(w1580) -> ()
              }
              frame "u" {
                n766 = Generate User Event(user event=w1581, event data cluster="ignoreaction: uco" ("event data")) -> ()  [unwired: 2 in, 2 out]
              }
              frame "p" {
                n767 = Generate User Event ("action User Event")(user event=w1584, event data cluster="action: copy to math" ("event data")) -> ()  [unwired: 2 in, 2 out]
              }
              frame "q" {
                n768 = Generate User Event ("action User Event")(user event=w1586, event data cluster="action: copy from math" ("event data")) -> ()  [unwired: 2 in, 2 out]
              }
              frame "\\", "|" {
                n769 = for {
                  N: 1 -> [_]
                  tunnel: w1590 -> [w1604]
                  tunnel: w1588 -> [w1603]
                  tunnel: [w1603] -> w1587
                  n770 = local read "selection :|\\"() -> (w1596:u16)
                  n771 = property on="selection :|\\" class="Ring (strict)"() -> ("NumItems"=w1594:u32)  [unwired: 2 in, 2 out]
                  n772 = To Long Integer(number=w1596) -> (32bit integer=w1595:i32)
                  n773 = case shown="\"|\", Default" w1604 {
                    tunnel: w1595 -> [w1606 w1608]
                    tunnel: [w1605 w1607] -> w1600
                    frame "|", Default {
                      n774 = Decrement(x=w1606) -> (x-1=w1605:i32)
                    }
                    frame "\\" {
                      n775 = Increment(x=w1608) -> (x+1=w1607:i32)
                    }
                  }
                  n776 = To Long Integer(number=w1594) -> (32bit integer=w1593:i32)
                  n777 = Greater Or Equal?(x=w1600, y=w1593) -> (x >= y?=w1602:bool)
                  n778 = Select(t=u16 0 ("lower limit"), s=w1602, f=w1600) -> (s? t:f=w1597:i32)
                  n779 = Decrement(x=w1593) -> (x-1=w1598:i32)
                  n780 = Less Than 0?(x=w1597) -> (x < 0?=w1599:bool)
                  n781 = Select(t=w1598, s=w1599, f=w1597) -> (s? t:f=w1592:i32)
                  n782 = local write "selection :|\\"(w1592) -> ()
                }
                n783 = Generate User Event ("action User Event")(user event=w1587, event data cluster="action: constrained filenames select" ("event data")) -> ()  [unwired: 2 in, 2 out]
              }
              frame "m" {
                n784 = Generate User Event ("action User Event")(user event=w1609, event data cluster="action: copy from math" ("event data")) -> ()  [unwired: 2 in, 2 out]
              }
            }
          }
          frame "PageUp" {
          }
          frame "Enter" {
            n785 = Generate User Event ("action User Event")(user event=w1611, event data cluster="action: new sweep" ("event data")) -> (user event out=w1612:refnum<user-event>)  [unwired: 2 in, 1 out]
            n786 = Generate User Event ("action User Event")(user event=w1612, event data cluster="action: replot colors" ("event data")) -> ()  [unwired: 2 in, 2 out]
          }
          frame "Caps" {
          }
          frame "PageDown" {
          }
          frame "Up".."Right" {
            n787 = case shown="\"Down\"" w1617 {
              tunnel: [cursor_action."zoom in 20%" ("cursor action") cursor_action."zoom out 20%" ("cursor action") cursor_action."zoom out 20%" ("cursor action") cursor_action."zoom in 20%" ("cursor action")] -> w1615
              frame "Up", Default {
              }
              frame "Down" {
              }
              frame "Left" {
              }
              frame "Right" {
              }
            }
            n788 = call "replace cursor - plot ref - V2.vi"("Plot ref in"=w1616, "cursor action"=w1615) -> ()  [unwired: 14 in, 4 out]
          }
        }
      }
      event Value Change {
        # "\"interface: update curvature plot\""
        n789 = event-data() -> ()  [unwired: 1 in, 6 out]
        n790 = Generate User Event(user event=w1622, event data cluster="interface: update curvature plot" ("event data")) -> ()  [unwired: 2 in, 2 out]
      }
      event "Plot:  colors": Cursor Move {
        (unwired) "interface: plot colors update m1m2m3 cursors" ("event data")
        n791 = event-data() -> ("CursIdx"=w1633:i32)  [unwired: 1 in]
        n792 = local read "reverse cursor index map"() -> (w1634:map{i32, T1})
